vi "Read-Save DefaultNotes.vi"(6 "Task":enum16{"Save", "Read"}(ring)=enum."Read", 11 "Notes":string) -> (0 "Pref Path":path, 3 "Notes Out":string)   [LabVIEW 2022 SP3]
panel:
  out "text":string
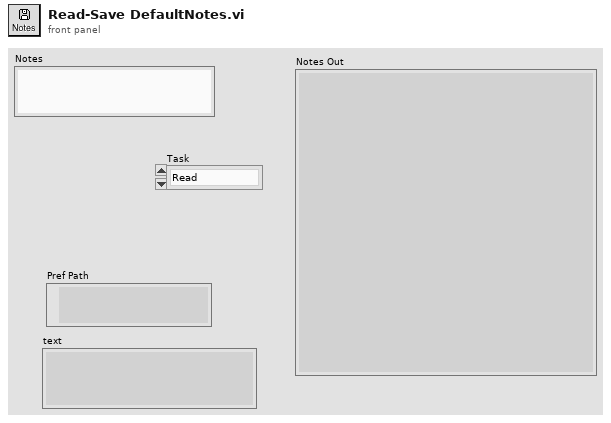
[diagram p1: front panel]
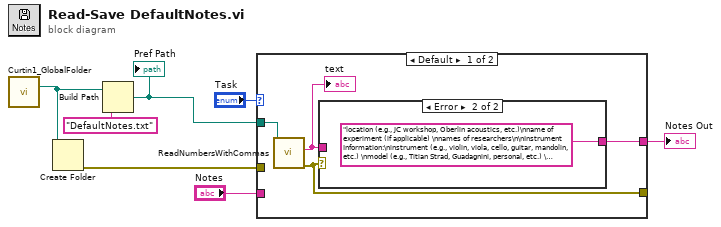
[diagram p0: block diagram]
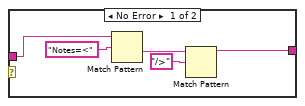
[diagram p2: hidden frame]
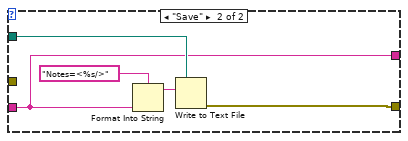
[diagram p3: hidden frame]
diagram:
  n1 = call "Curtin1_GlobalFolder.vi"() -> ("LabVIEW Data Path"=w1:path)  [unwired: 1 in, 1 out]
  n2 = Create Folder(path (use dialog)=w1) -> (error out=w2:errorcluster)  [unwired: 2 in, 2 out]
  n3 = Build Path(base path=w1, name or relative path="DefaultNotes.txt") -> (appended path=w6:path)
  "Pref Path" <- w6
  n4 = case shown="Default" "Task" {
    tunnel: "Notes" -> [_ w18]
    tunnel: w6 -> [w10 w22]
    tunnel: [w8 w19] -> _
    tunnel: [w11 w18] -> w3
    tunnel: w2 -> [_ _]
    frame Default {
      n5 = call "ReadNumbersWithCommas.vi"("file (use dialog)"=w10) -> ("error out"=w8:errorcluster, "text"=w9:string)  [unwired: 7 in, 2 out]
      "text" <- w9
      n6 = case shown="Error" w8 {
        tunnel: [w12 "location (e.g., JC workshop, Oberlin acoustics, etc.)\nname of experiment (if applicable) \nnames of researchers\n\nInstrument Information:\ninstrument (e.g., violin, viola, cello, guitar, mandolin, etc.) \nmodel (e.g., Titian Strad, Guadagnini, personal, etc.) \nmaker name\nmaker ID (e.g., serial number)\nyear built (4 digits)\ncountry of origin \nsession (e.g. Oberlin 2017, VSA 2008) \nmaking school (e.g. Old Italian) \n\nMeasurement Information:\ntype (Radiation, admittance, modal analysis, taptones, etc.) \nprotocol (HV24, etc.)\n" ("Notes")] -> w11
        tunnel: w9 -> [w16 _]
        frame No Error {
          n7 = Match Pattern(string=w16, regular expression="Notes=<" ("format string")) -> (after substring=w15:string)  [unwired: 1 in, 3 out]
          n8 = Match Pattern(string=w15, regular expression="/>" ("format string")) -> (before substring=w12:string)  [unwired: 1 in, 3 out]
        }
        frame Error {
        }
      }
    }
    frame "Save" {
      n9 = Format Into String(format string="Notes=<%s/>", w18) -> (resulting string=w21:string)  [unwired: 2 in, 1 out]
      n10 = Write to Text File(file (use dialog)=w22, text=w21) -> (error out=w19:errorcluster)  [unwired: 2 in, 2 out]
    }
  }
  "Notes Out" <- w3
